vi "cluster error.vi"() -> ()   [LabVIEW 2018]
panel:
  in  "Numeric 2":dbl
  out "Numeric":dbl
  out "error out":errorcluster
  in  "error in (no error)":errorcluster
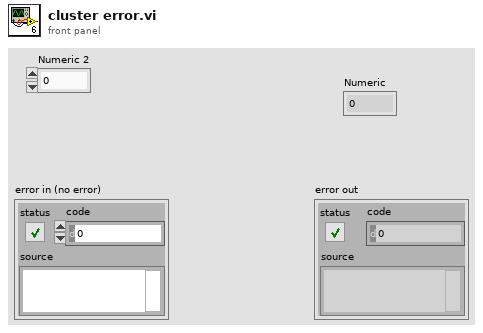
[diagram p1: front panel]
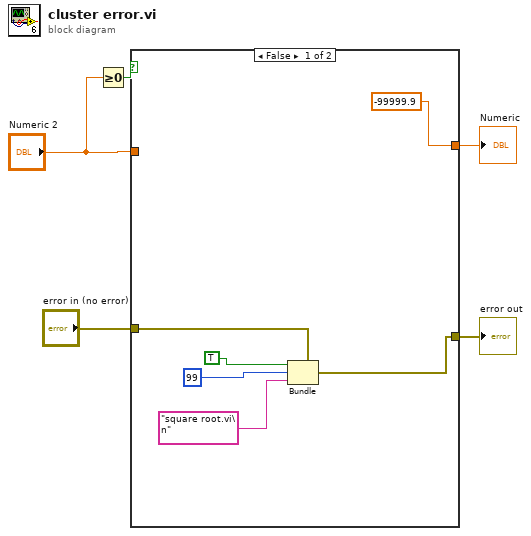
[diagram p0: block diagram]
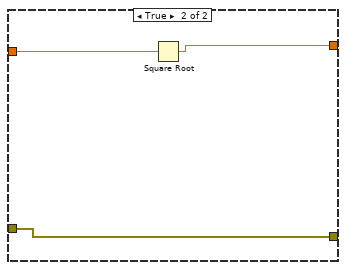
[diagram p2: hidden frame]
diagram:
  n1 = Greater Or Equal To 0?(x="Numeric 2") -> (x >= 0?=w4:bool)
  n2 = case shown="False" w4 {
    tunnel: "Numeric 2" -> [_ w14]
    tunnel: [-99999.9 w13] -> w5
    tunnel: "error in (no error)" -> [w10 w12]
    tunnel: [w9 w12] -> w1
    frame False {
      n3 = Bundle(cluster=w10, "status"=TRUE, "code"=99, "source"="square root.vi\n") -> (w9:errorcluster)
    }
    frame True {
      n4 = Square Root(x=w14) -> (sqrt(x)=w13:dbl)
    }
  }
  "error out" <- w1
  "Numeric" <- w5
